vi "TrianglesSym.vi"(10 "Rotation":T1, 11 "TrianglesIn":T2[](array[typedef])) -> (3 "TrianglesOut":T2[](array[typedef]))   [LabVIEW 2014]
uses:
  TypeDefs/TriangleFace.ctl
  TypeDefs/Point3D.ctl
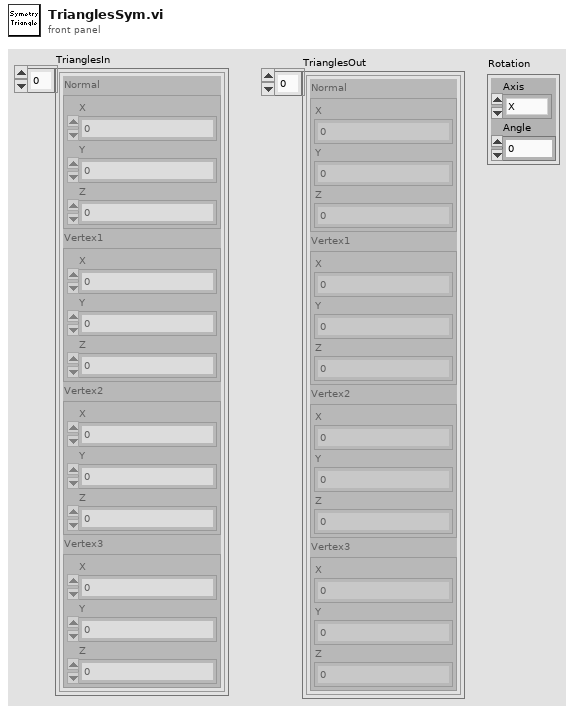
[diagram p1: front panel]
types:
  T1 = cluster{"Axis":enum16{"X", "Y", "Z"}, "Angle":sgl}
  T2 = typedef "TriangleFace.ctl" = cluster{"Normal":T3, "Vertex1":T3, "Vertex2":T3, "Vertex3":T3}
  T3 = typedef "Point3D.ctl" = cluster{"X":sgl, "Y":sgl, "Z":sgl}
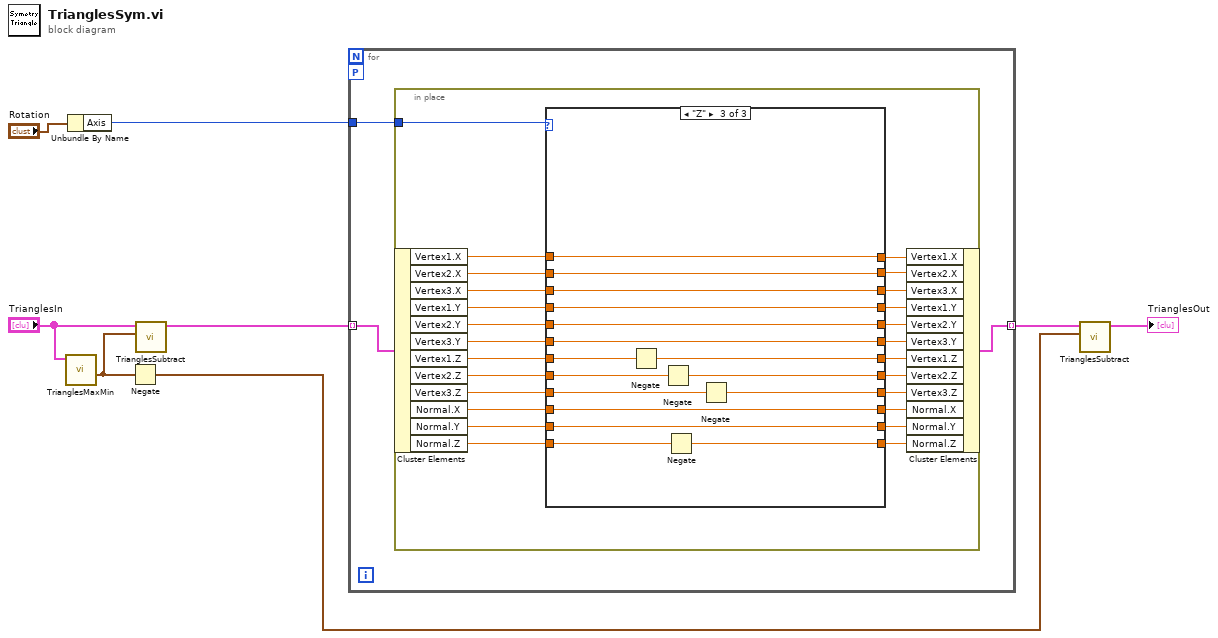
[diagram p0: block diagram]
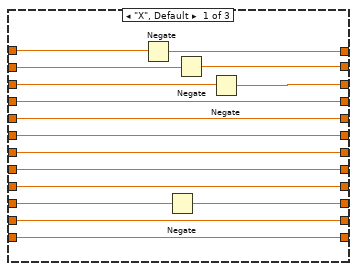
[diagram p2: hidden frame]
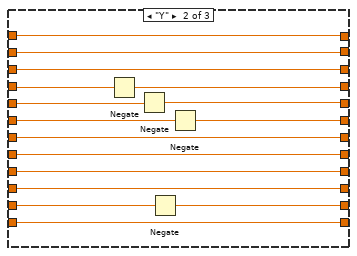
[diagram p3: hidden frame]
diagram:
  n1 = call "TrianglesMaxMin.vi"("Triangles"="TrianglesIn") -> ("Center"=w5:T3)  [unwired: 8 in, 2 out]
  n2 = Unbundle By Name("Rotation") -> ("Axis"=w1:enum16{"X", "Y", "Z"})
  n3 = Negate(x=w5) -> (-x=w4:T3)
  n4 = call "TrianglesSubtract.vi"("Point3D"=w5, "TrianglesIn"="TrianglesIn") -> ("TrianglesOut"=w7:T2[])  [unwired: 9 in]
  n5 = for {
    tunnel: w7 -> [w11] mode=indexing
    tunnel: [w10] -> w6 mode=indexing
    workers-P: _ -> [_]
    tunnel: w1 -> [w9]
    n6 = in-place {
      in-place-border: w9 -> [w36]
      n7 = in-place-cluster #1(w11) -> ("Vertex1.X"=w19:sgl, "Vertex2.X"=w17:sgl, "Vertex3.X"=w15:sgl, "Vertex1.Y"=w34:sgl, "Vertex2.Y"=w32:sgl, "Vertex3.Y"=w30:sgl, "Vertex1.Z"=w28:sgl, "Vertex2.Z"=w26:sgl, "Vertex3.Z"=w24:sgl, "Normal.X"=w13:sgl, "Normal.Y"=w22:sgl, "Normal.Z"=w20:sgl)
      n8 = case shown="\"Z\"" w36 {
        tunnel: [w52 w59 w81] -> w35
        tunnel: w34 -> [w52 w60 w81]
        tunnel: [w51 w57 w80] -> w33
        tunnel: w32 -> [w51 w58 w80]
        tunnel: [w50 w55 w79] -> w31
        tunnel: w30 -> [w50 w56 w79]
        tunnel: [w49 w65 w75] -> w29
        tunnel: w28 -> [w49 w65 w76]
        tunnel: [w48 w64 w73] -> w27
        tunnel: w26 -> [w48 w64 w74]
        tunnel: [w47 w63 w71] -> w25
        tunnel: w24 -> [w47 w63 w72]
        tunnel: [w46 w53 w77] -> w23
        tunnel: w22 -> [w46 w54 w77]
        tunnel: [w45 w62 w69] -> w21
        tunnel: w20 -> [w45 w62 w70]
        tunnel: w19 -> [w44 w68 w84]
        tunnel: [w43 w68 w84] -> w18
        tunnel: w17 -> [w42 w67 w83]
        tunnel: [w41 w67 w83] -> w16
        tunnel: w15 -> [w40 w66 w82]
        tunnel: [w39 w66 w82] -> w14
        tunnel: w13 -> [w38 w61 w78]
        tunnel: [w37 w61 w78] -> w12
        frame "X", Default {
          n9 = Negate(x=w44) -> (-x=w43:sgl)
          n10 = Negate(x=w38) -> (-x=w37:sgl)
          n11 = Negate(x=w42) -> (-x=w41:sgl)
          n12 = Negate(x=w40) -> (-x=w39:sgl)
        }
        frame "Y" {
          n13 = Negate(x=w60) -> (-x=w59:sgl)
          n14 = Negate(x=w58) -> (-x=w57:sgl)
          n15 = Negate(x=w54) -> (-x=w53:sgl)
          n16 = Negate(x=w56) -> (-x=w55:sgl)
        }
        frame "Z" {
          n17 = Negate(x=w76) -> (-x=w75:sgl)
          n18 = Negate(x=w74) -> (-x=w73:sgl)
          n19 = Negate(x=w70) -> (-x=w69:sgl)
          n20 = Negate(x=w72) -> (-x=w71:sgl)
        }
      }
      n21 = in-place-cluster #1("Vertex1.X"=w18, "Vertex2.X"=w16, "Vertex3.X"=w14, "Vertex1.Y"=w35, "Vertex2.Y"=w33, "Vertex3.Y"=w31, "Vertex1.Z"=w29, "Vertex2.Z"=w27, "Vertex3.Z"=w25, "Normal.X"=w12, "Normal.Y"=w23, "Normal.Z"=w21) -> (w10:T2)
    }
  }
  n22 = call "TrianglesSubtract.vi"("Point3D"=w4, "TrianglesIn"=w6) -> ("TrianglesOut"=→"TrianglesOut":T2[])  [unwired: 9 in]
